vi "Slice Usage Test.vi"() -> ()   [LabVIEW 2019]
uses:
  SPI/SPI Config.ctl
panel:
  out "Gyro Data":T1
  out "Accelerometer Data":T1
  out "SPI Config Out":T2
  out "Data Out 2":T3
  out "Data Out":T4 {"ID" format="%x"}
  in  "Control Value":fxp<+/-,32,16>
  in  "ID":u32 format="%x"
  in  "SPI Config In":T2
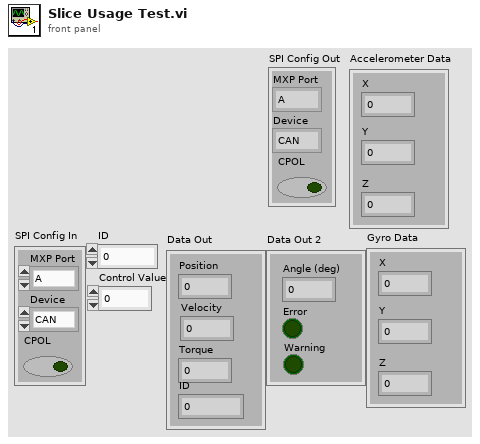
[diagram p1: front panel]
types:
  T1 = cluster{fxp<+/-,32,16>, fxp<+/-,32,16>, fxp<+/-,32,16>}
  T2 = typedef "SPI Config.ctl" = cluster{"MXP Port":enum16{"A", "B"}, "Device":enum16{"CAN", "ENC", "IMU1", "IMU2"}, "CPOL":bool}
  T3 = cluster{"Angle (deg)":fxp<+/-,64,32>, "Error":bool, "Warning":bool}
  T4 = cluster{"Position":fxp<+/-,32,16>, "Velocity":fxp<+/-,32,16>, "Torque":fxp<+/-,32,16>, "ID":u32}
  T5 = cluster{"Angle (deg)":fxp<+,32,16>, "Error":bool, "Warning":bool}
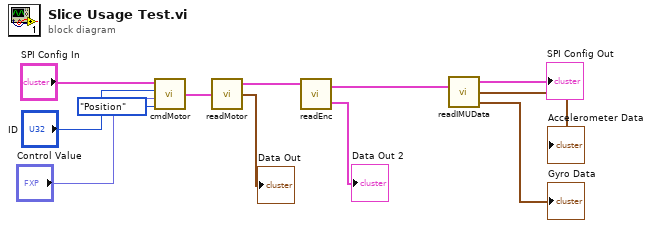
[diagram p0: block diagram]
diagram:
  n1 = call "cmdMotor.vi"("Mode"=enum16{"Position", "Velocity", "Torque"}."Position", "Control Value"="Control Value", "ID"="ID", "SPI Config In"="SPI Config In") -> ("SPI Config Out"=w12:T2)
  n2 = call "readMotor.vi"("SPI Config In"=w12) -> ("SPI Config Out"=w7:T2, "Data Out"=→"Data Out":T4)  [unwired: 1 out]
  n3 = call "readEnc.vi"("SPI Config In"=w7) -> ("SPI Config Out"=w4:T2, "Data Out"=→"Data Out 2":T5)
  n4 = call "readIMUData.vi"("SPI Config In"=w4) -> ("SPI Config Out"=→"SPI Config Out":T2, "Accelerometer Data"=→"Accelerometer Data":T1, "Gyro Data"=→"Gyro Data":T1)  [unwired: 1 in]
